vi "Prepare - Initialize Objects.vi"(7 "Buttons Def File":path, 8 "error in (no error)":errorcluster, 9 "Pane":refnum<vi>, 11 "Control Refs":T1) -> (0 "error out":errorcluster, 2 "HSE VBox Layout":refnum<class "HSE VBoxLayout.lvclass">, 3 "Button Manager out":refnum<class "Button Manager.lvclass">)   [LabVIEW 2022 SP3, in "Navigation.lvlib"]
doc: "____\nHAMPEL SOFTWARE ENGINEERING v2.6.0 (2023-12-19 10:54)"
uses:
  Navigation.lvlib
  Button Manager/Control Refs.ctl
  Button Manager/Button Manager.lvclass
  <vilib>/Hampel Software Engineering/HSE Layout Manager/HSE Layout/HSE VBoxLayout/HSE VBoxLayout.lvclass
  <vilib>/Utility/miscctls.llb/LVPointTypeDef.ctl
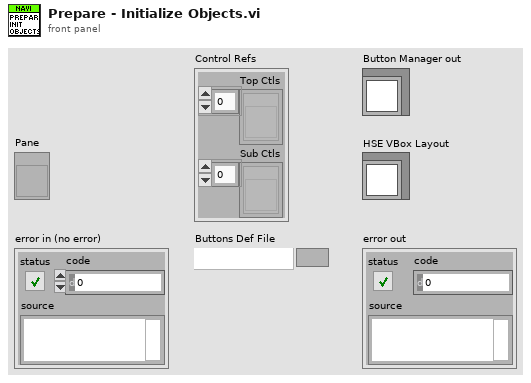
[diagram p1: front panel]
types:
  T1 = typedef "Navigation.lvlib/Button Manager.lvclass/Control Refs.ctl" = cluster{"Top Ctls":refnum<vi>[], "Sub Ctls":refnum<vi>[]}
  T2 = typedef "LVPointTypeDef.ctl" = cluster{"Horizontal":i16, "Vertical":i16}
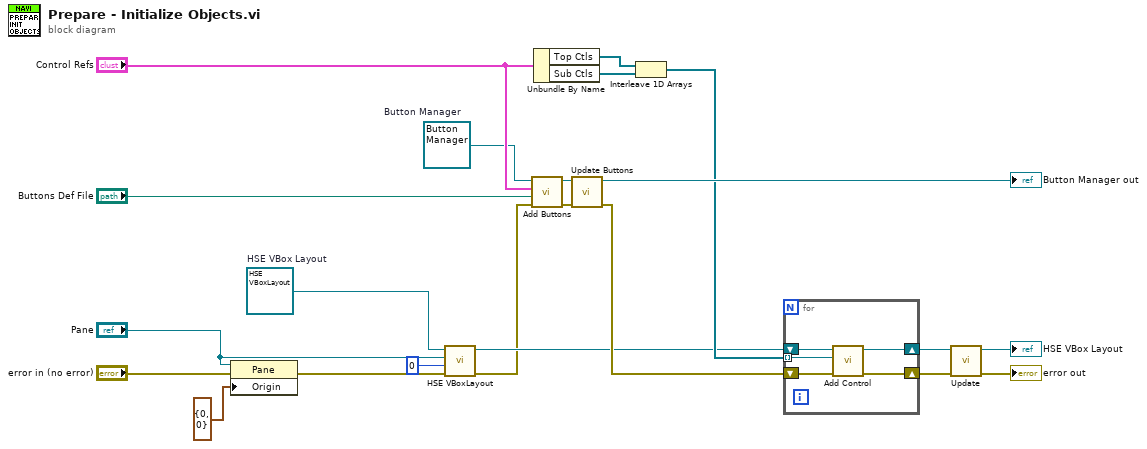
[diagram p0: block diagram]
diagram:
  w1 = refnum<class "HSE VBoxLayout.lvclass"> refnum  # HSE VBox Layout
  w16 = refnum<class "Button Manager.lvclass"> refnum  # Button Manager
  n1 = property on="Property Node" class="Pane"(reference="Pane", error in="error in (no error)", "Origin"=T2 {"Horizontal"=0, "Vertical"=0}) -> (error out=w8:errorcluster)  [unwired: 1 out]
  n2 = call-dynamic "HSE VBoxLayout.vi"("error in"=w8, "Spacing"=0, "Parent Pane"="Pane", "HSE VBoxLayout"=w1) -> ("error out"=w5:errorcluster, "HSE VBoxLayout out"=w9:refnum<class "HSE VBoxLayout.lvclass">)  [unwired: 6 in]
  n3 = call-dynamic "Add Buttons.vi"("error in"=w5, "Button Def JSON"="Buttons Def File", "Control Refs"="Control Refs", "Button Manager in"=w16) -> ("error out"=w11:errorcluster, "Button Manager out"=w12:refnum<class "Button Manager.lvclass">)  [unwired: 6 in]
  n4 = Unbundle By Name("Control Refs") -> ("Top Ctls"=w13:refnum<vi>[], "Sub Ctls"=w14:refnum<vi>[])
  n5 = call-dynamic "Update Buttons.vi"("error in"=w11, "Button Manager in"=w12) -> ("error out"=w10:errorcluster, "Button Manager out"=→"Button Manager out":refnum<class "Button Manager.lvclass">)  [unwired: 8 in]
  n6 = Interleave 1D Arrays(w13, w14) -> (w15:refnum<vi>[])
  n7 = for {
    shift-right: [w25] -> w2
    shift-left: w9 -> [w27]
    shift-right: [w24] -> w3
    shift-left: w10 -> [w26]
    tunnel: w15 -> [w23] mode=indexing
    n8 = call-dynamic "Add Control.vi"("error in"=w26, "Ctl Refnum"=w23, "HSE Layout in"=w27) -> ("error out"=w24:errorcluster, "HSE Layout out"=w25:refnum<class "HSE VBoxLayout.lvclass">)  [unwired: 7 in]
  }
  n9 = call-dynamic "Update.vi"("error in"=w3, "HSE VBoxLayout in"=w2) -> ("error out"=→"error out":errorcluster, "HSE VBoxLayout out"=→"HSE VBox Layout":refnum<class "HSE VBoxLayout.lvclass">)  [unwired: 8 in]
